vi "Intacc Teleop.vi"(9 "Joystick Buttons":bool[](array[boolean]), 11 "Axes":dbl[](array[numeric])) -> ()   [LabVIEW 2019]
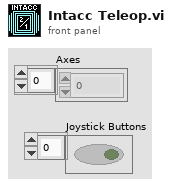
[diagram p1: front panel]
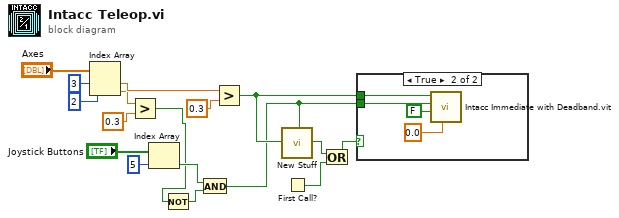
[diagram p0: block diagram]
diagram:
  n1 = Index Array(array="Axes", index #1=3 ("index"), index #2=2 ("index")) -> (element #1=w15:dbl, element #2=w5:dbl)
  n2 = Greater?(x=w5, y=0.3) -> (0:w4:bool)
  n3 = Index Array(array="Joystick Buttons", index=5) -> (element=w10:bool)
  n4 = Not(x=w4) -> (.not. x?=w9:bool)
  n5 = And(x=w10, y=w9) -> (x .and. y?=w8:bool)
  n6 = Greater?(x=w15, y=0.3) -> (0:w13:bool)
  n7 = call "New Stuff.vi"("Variant 3"=w13, "Variant 10"=w8) -> ("x != y?"=w3:bool)  [unwired: 25 in]
  n8 = First Call?() -> (First Call?: T/F=w1:bool)
  n9 = Or(x=w3, y=w1) -> (x .or. y?=w2:bool)
  n10 = case shown="True" w2 {
    tunnel: w13 -> [_ w21]
    tunnel: w8 -> [_ w20]
    frame False {
    }
    frame True {
      n11 = call "Intacc Immediate with Deadband.vit"("Position to override"=0.0, "Override position?"=FALSE, "Reverse?"=w20, "Intaking?"=w21) -> ()  [unwired: 7 in, 1 out]
    }
  }
